vi "checkTempConfig.vi"(8 "ERROR IN":errorcluster) -> (0 "ERROR OUT":errorcluster, 1 "tempConfigIsOk?":bool=TRUE, 3 "tempConfig":T1={"ComPort"="COM4", "SensorNumber"=1.0, "PID"={"P"=0.0, "I"=0.0, "D"=0.0}})   [LabVIEW 2020]
uses:
  defTypeConfigs/tempConfig.ctl
  var globales/closeThreads.vi
panel:
  out "DAQ 2":dbl
  out "DAQ 1":dbl
  out "Luxtron 1":dbl
  out "temps":dbl
  in  "Stop acquisition":bool
  out "Luxtron 2":dbl
  in  "Consigne":dbl
  out "Graphe XY":cluster{"X":dbl[], "Y":dbl[]}[](graph)
  in  "Select Serial Port":refnum<visa-resource-name>="COM1"
  # "Temperature sensor \nconfiguration"
  # "COM port heat sensor\nHeat sensor number\nPID configuration"
  # "PID configuration"
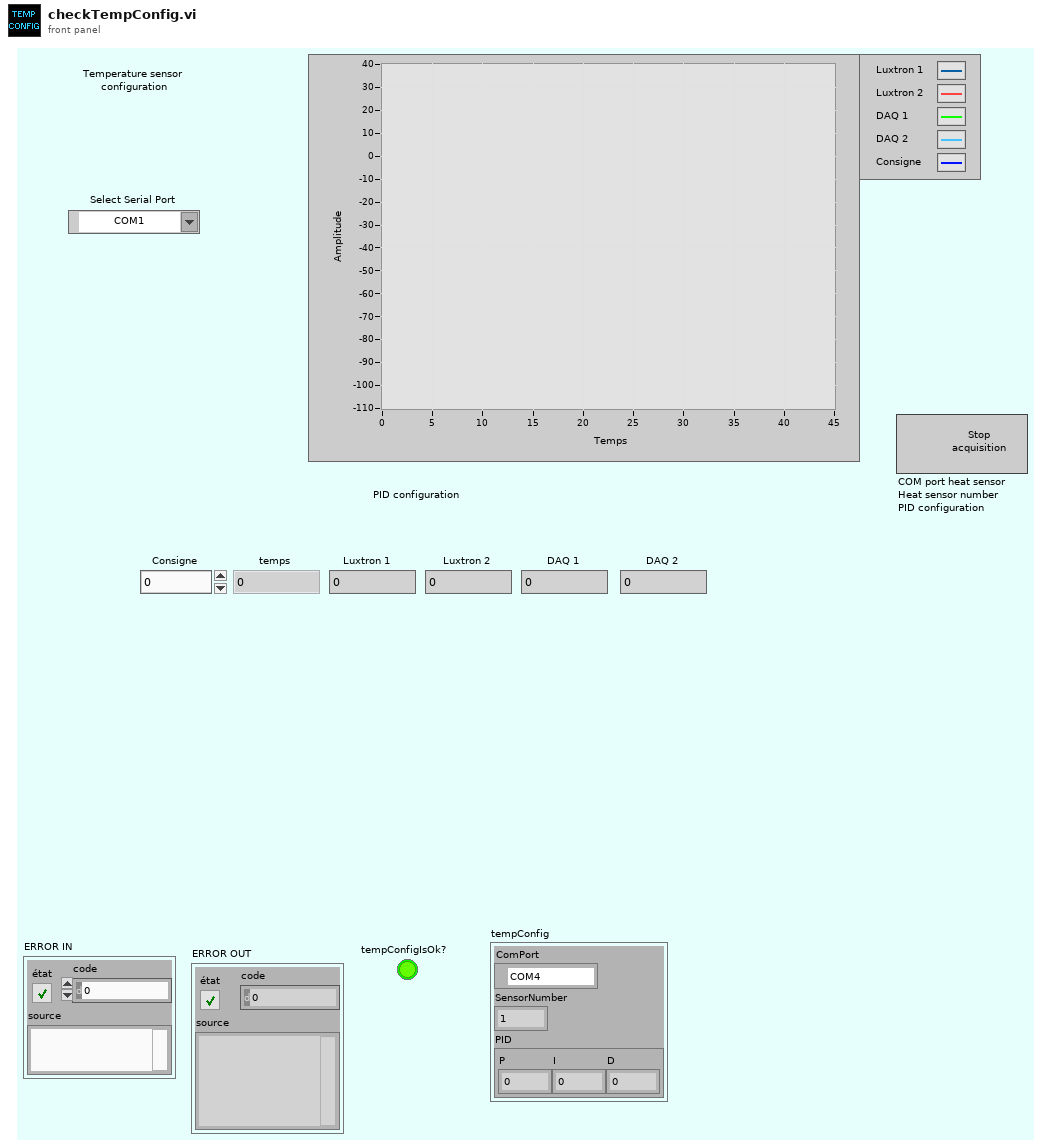
[diagram p1: front panel]
types:
  T1 = typedef "tempConfig.ctl" = cluster{"ComPort":refnum<visa-resource-name>, "SensorNumber":dbl, "PID":cluster{"P":dbl, "I":dbl, "D":dbl}}
  T2 = cluster{"sensor Luxtron1":dbl, "sensor Luxtron2":dbl, "sensor DAQ1":dbl, "sensor DAQ2":dbl, "temps":dbl}
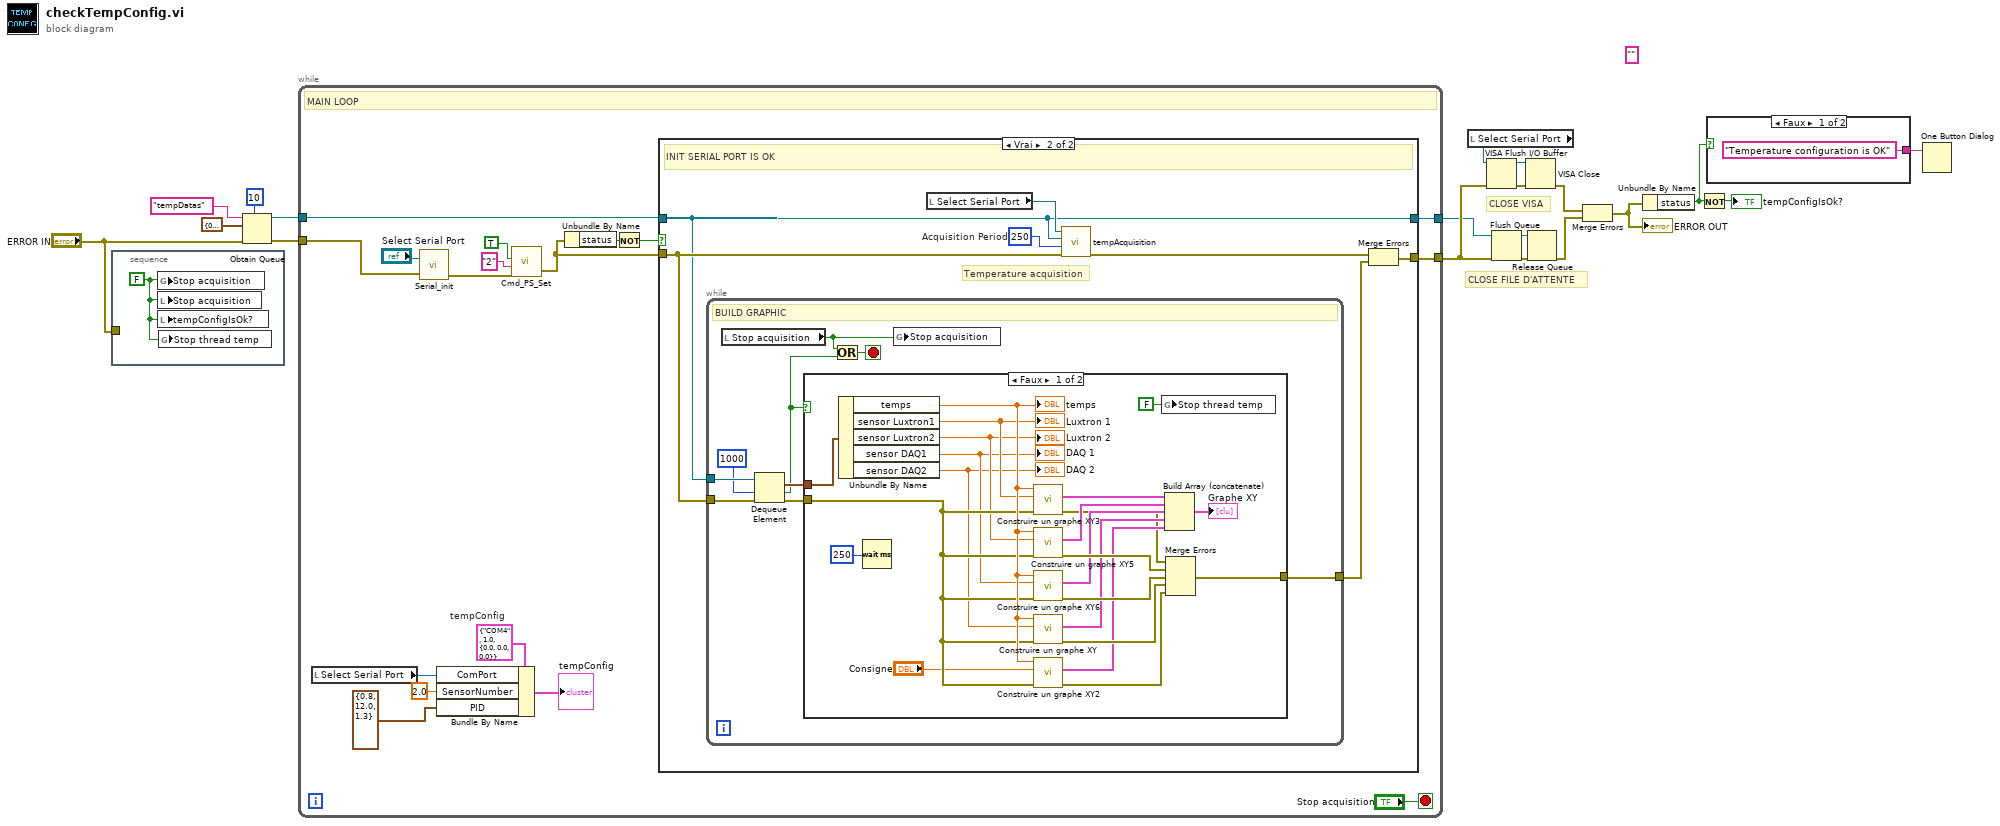
[diagram p0: block diagram]
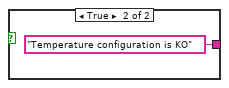
[diagram p2: hidden frame]
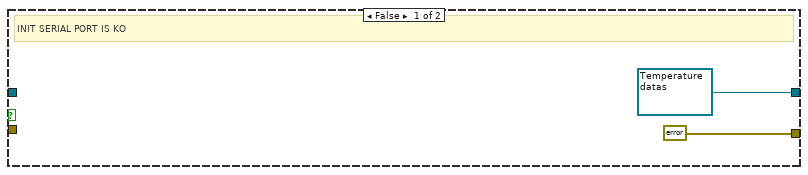
[diagram p3: hidden frame]
diagram:
  (unwired) "" ("message")
  # "CLOSE FILE D'ATTENTE"
  # "CLOSE VISA"
  n1 = stacked-sequence {
    tunnel: "ERROR IN" -> [_]
    frame #0 {
      w20 = FALSE
      n2 = global write "closeThreads.vi" "Stop acquisition"(w20) -> ()
      n3 = local write "Stop acquisition"(w20) -> ()
      n4 = local write "tempConfigIsOk?"(w20) -> ()
      n5 = global write "closeThreads.vi" "Stop thread temp"(w20) -> ()
    }
  }
  n6 = Obtain Queue(max queue size (-1, unlimited)=10 ("taille max de la file d'attente (-1, non limitée)"), name (unnamed)="tempDatas" ("nom (aucun)"), element data type=T2 {"sensor Luxtron1"=0.0, "sensor Luxtron2"=36.42, "sensor DAQ1"=0.0, "sensor DAQ2"=0.0, "temps"=122.90212535858154} ("Temperature datas"), error in (no error)="ERROR IN") -> (queue out=w5:refnum<queue>, error out=w4:errorcluster)  [unwired: 1 in, 1 out]
  n7 = while {
    tunnel: [w25] -> w10
    tunnel: [w26] -> w13
    tunnel: w5 -> [w24]
    tunnel: w4 -> [w23]
    stop <- "Stop acquisition" stop-if-true
    w29 = T1 {"ComPort"="COM4", "SensorNumber"=1.0, "PID"={"P"=0.0, "I"=0.0, "D"=0.0}}  # tempConfig
    # "MAIN LOOP"
    n8 = local read "Select Serial Port"() -> (w27:refnum<visa-resource-name>)
    n9 = call "Serial_init.vi"("VISA resource name"="Select Serial Port", "error IN"=w23) -> ("error OUT"=w34:errorcluster)  [unwired: 2 out]
    n10 = Bundle By Name(cluster=w29, "ComPort"=w27, "SensorNumber"=2.0, "PID"=cluster{"P":dbl, "I":dbl, "D":dbl} {"P"=0.8, "I"=12.0, "D"=1.3}) -> (→"tempConfig":T1)
    n11 = call "Cmd_PS_Set.vi"("error IN"=w34, "Write String"="2", "Send Command"=TRUE) -> ("error out"=w22:errorcluster)  [unwired: 1 in, 1 out]
    n12 = Unbundle By Name(w22) -> ("status"=w33:bool)
    n13 = Not(x=w33) -> (.not. x?=w32:bool)
    n14 = case shown="Vrai" w32 {
      tunnel: w22 -> [_ w45]
      tunnel: [errorcluster {"status"=TRUE, "code"=0, "source"=""} ("error IO") w43] -> w26
      tunnel: [refnum<queue> refnum ("file d'attente") w41] -> w25
      tunnel: w24 -> [_ w41]
      frame False {
        # "INIT SERIAL PORT IS KO"
      }
      frame True {
        w46 = u32 250  # Acquisition Period
        # "Temperature acquisition"
        # "INIT SERIAL PORT IS OK"
        n15 = while {
          tunnel: w45 -> [w52]
          tunnel: [w55] -> w42
          tunnel: w41 -> [w51]
          stop <- w48 stop-if-true
          # "BUILD GRAPHIC"
          n16 = local read "Stop acquisition"() -> (w47:bool)
          n17 = Dequeue Element(queue=w51, timeout in ms (-1)=1000 ("timeout en ms (-1)"), error in (no error)=w52) -> (element=w54:T2, timed out?=w49:bool, error out=w53:errorcluster)  [unwired: 1 out]
          n18 = case shown="Faux" w49 {
            tunnel: [w74 w78] -> w55
            tunnel: w54 -> [w71 _]
            tunnel: w53 -> [w65 w78]
            frame False {
              n19 = Unbundle By Name(w71) -> ("temps"=w66:dbl, "sensor Luxtron1"=w63:dbl, "sensor Luxtron2"=w62:dbl, "sensor DAQ1"=w61:dbl, "sensor DAQ2"=w60:dbl)
              "Luxtron 2" <- w62
              "temps" <- w66
              "Luxtron 1" <- w63
              "DAQ 2" <- w60
              "DAQ 1" <- w61
              n20 = Wait (ms)(milliseconds to wait=u32 250 ("attente (ms)")) -> ()  [unwired: 1 out]
              n21 = call "Construire un graphe XY3"("error in (no error)"=w65, "Y Input"=w63, "X Input"=w66) -> ("error out"=w58:errorcluster, "XY Graph"=w64:cluster{"X":dbl[], "Y":dbl[]}[])  [unwired: 7 in]
              n22 = call "Construire un graphe XY5"("error in (no error)"=w65, "Y Input"=w62, "X Input"=w66) -> ("error out"=w76:errorcluster, "XY Graph"=w73:cluster{"X":dbl[], "Y":dbl[]}[])  [unwired: 7 in]
              n23 = call "Construire un graphe XY6"("error in (no error)"=w65, "Y Input"=w61, "X Input"=w66) -> ("error out"=w75:errorcluster, "XY Graph"=w72:cluster{"X":dbl[], "Y":dbl[]}[])  [unwired: 7 in]
              n24 = call "Construire un graphe XY"("error in (no error)"=w65, "Y Input"=w60, "X Input"=w66) -> ("error out"=w70:errorcluster, "XY Graph"=w68:cluster{"X":dbl[], "Y":dbl[]}[])  [unwired: 7 in]
              n25 = call "Construire un graphe XY2"("error in (no error)"=w65, "Y Input"="Consigne", "X Input"=w66) -> ("error out"=w69:errorcluster, "XY Graph"=w67:cluster{"X":dbl[], "Y":dbl[]}[])  [unwired: 7 in]
              n26 = global write "closeThreads.vi" "Stop thread temp"(FALSE ("Stop thread temp")) -> ()
              n27 = Build Array (concatenate)(w64, w73, w72, w68, w67) -> (→"Graphe XY":cluster{"X":dbl[], "Y":dbl[]}[])
              n28 = Merge Errors(w58, w76, w75, w70, w69) -> (w74:errorcluster)
            }
            frame True {
            }
          }
          n29 = Or(x=w47, y=w49) -> (x .or. y?=w48:bool)
          n30 = global write "closeThreads.vi" "Stop acquisition"(w47) -> ()
        }
        n31 = local read "Select Serial Port"() -> (w44:refnum<visa-resource-name>)
        n32 = call "tempAcquisition.vi"("Error IN"=w45, "Acquisition Period"=w46, "queue IN"=w41, "VISA"=w44) -> ("Error OUT"=w40:errorcluster)  [unwired: 7 in]
        n33 = Merge Errors(w40, w42) -> (w43:errorcluster)
      }
    }
  }
  n34 = local read "Select Serial Port"() -> (w17:refnum<visa-resource-name>)
  n35 = VISA Flush I/O Buffer(VISA resource name=w17, error in (no error)=w13) -> (VISA resource name out=w19:refnum<visa-resource-name>, error out=w18:errorcluster)  [unwired: 1 in]
  n36 = Flush Queue(queue=w10, error in (no error)=w13) -> (queue out=w16:refnum<queue>, error out=w15:errorcluster)  [unwired: 1 out]
  n37 = VISA Close(VISA resource name=w19, error in (no error)=w18) -> (error out=w12:errorcluster)
  n38 = Release Queue(queue=w16, error in (no error)=w15) -> (error out=w11:errorcluster)  [unwired: 1 in, 2 out]
  n39 = Merge Errors(w12, w11) -> (w9:errorcluster)
  "ERROR OUT" <- w9
  n40 = Unbundle By Name(w9) -> ("status"=w2:bool)
  n41 = Not(x=w2) -> (.not. x?=→"tempConfigIsOk?":bool)
  n42 = case shown="Faux" w2 {
    tunnel: ["Temperature configuration is OK" ("message") "Temperature configuration is KO" ("message")] -> w1
    frame False {
    }
    frame True {
    }
  }
  n43 = One Button Dialog ("Boîte de dialogue à un bouton")(message=w1) -> ()  [unwired: 1 in, 1 out]
